vi "Write Sonde Data cells to excel.vi"(0 "NI_report in":refnum<class "NI_report.lvclass">, 1 "milliseconds to wait":u32, 2 "all rows":string[][](array[string]), 3 "Row Offset In":i32=14, 5 "error in (no error)":errorcluster, 6 "Worksheet Names":string[](array[string]), 7 "Sample Array":i32[](array[numeric]), 9 "Sample Row \nBreak points":i32[](array[numeric]), 11 "Number of Sample Sheets":i32) -> (14 "NI_report out":refnum<class "NI_report.lvclass">, 16 "Row Offset Out":i32, 19 "error out":errorcluster)   [LabVIEW 2016]
uses:
  <vilib>/Utility/NIReport.llb/NI_report.lvclass
panel:
  out "Row Offset":i32
  out "sample subarray":string[][](array[string])
  out "Length":i32
  out "Breakpoint size":i32
  out "number of rows":i32
  out "size(s)":i32[](array[numeric])
  out "Current Sample Sheet":string
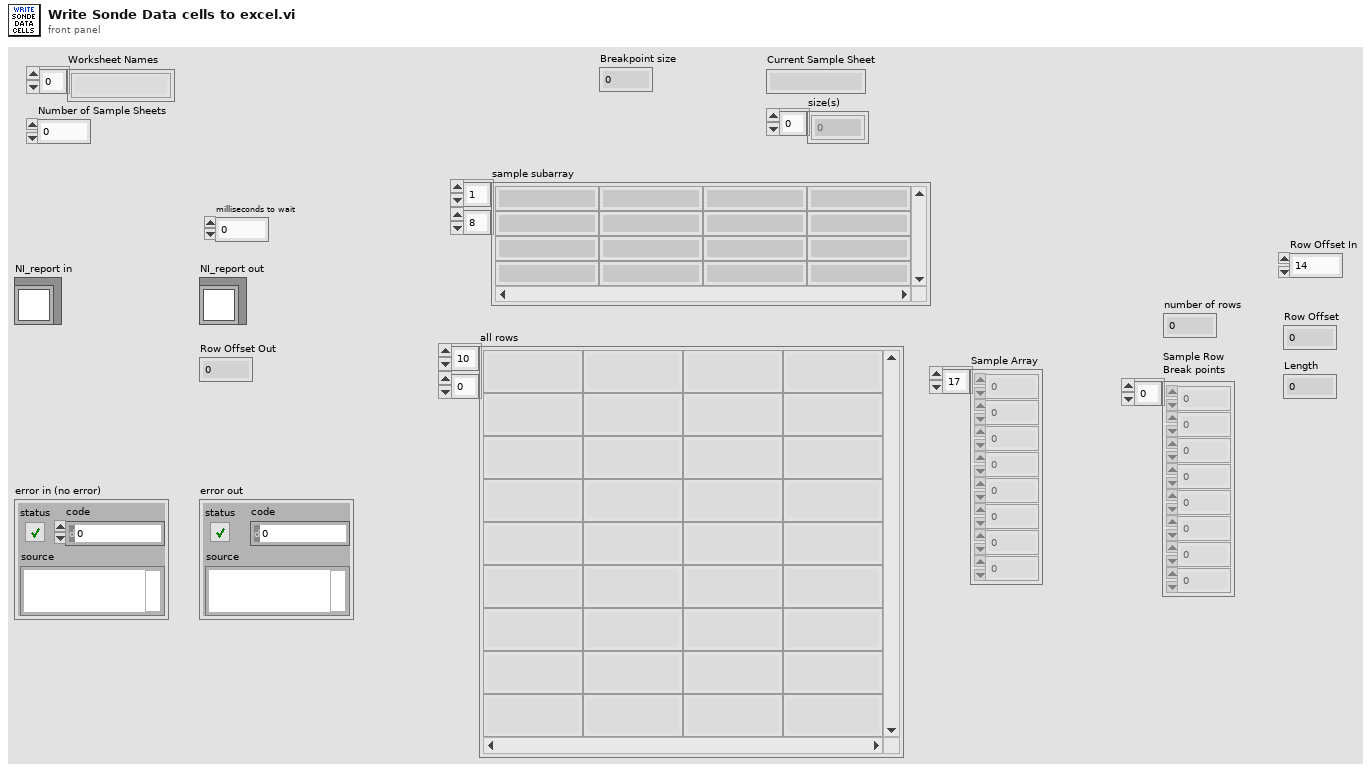
[diagram p1: front panel]
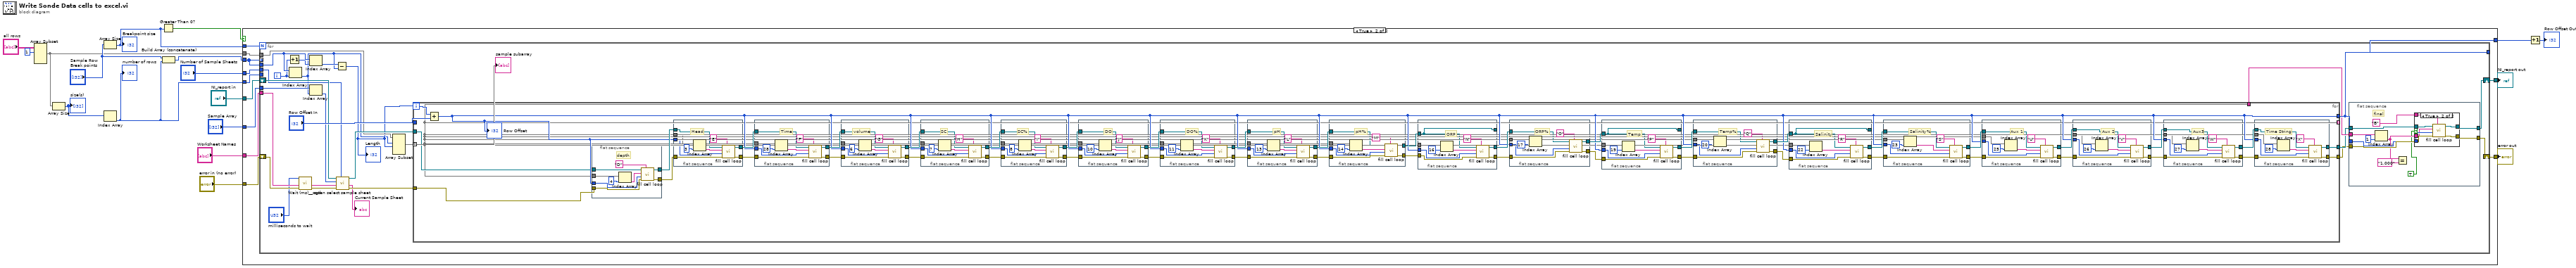
[diagram p0: block diagram]
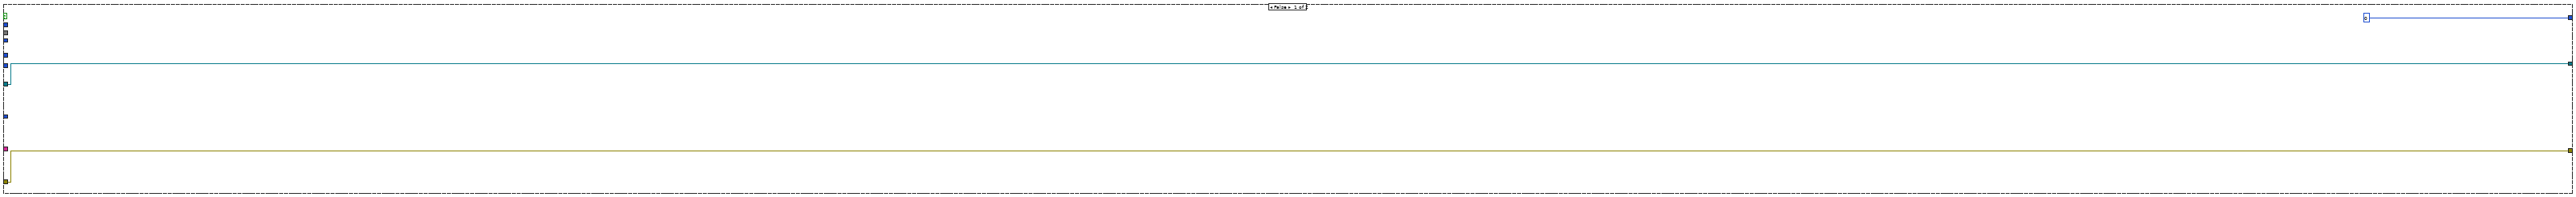
[diagram p2: hidden frame]
diagram:
  n1 = Array Subset(array="all rows", index (row)=1 ("index")) -> (w4:string[][])  [unwired: 3 in]
  n2 = Array Size(array=w4) -> (size(s)=w3:i32[])
  "size(s)" <- w3
  n3 = Array Size(array="Sample Row \nBreak points") -> (size(s)=w11:i32)
  "Breakpoint size" <- w11
  n4 = Index Array(array=w3) -> (element=w1:i32)  [unwired: 1 in]
  "number of rows" <- w1
  n5 = Greater Than 0?(x=w11) -> (x > 0?=w12:bool)
  n6 = Build Array (concatenate)("Sample Row \nBreak points", w1) -> (w2:i32[])
  n7 = case shown="True" w12 {
    tunnel: [w20 w33] -> w18
    tunnel: [w21 w32] -> w17
    tunnel: [0 ("Row Offset In") w31] -> w16
    tunnel: "NI_report in" -> [w21 w30]
    tunnel: "error in (no error)" -> [w20 w29]
    tunnel: w11 -> [_ w28]
    tunnel: w2 -> [_ w23]
    tunnel: "Sample Array" -> [_ w22]
    tunnel: "Worksheet Names" -> [_ w27]
    tunnel: "Number of Sample Sheets" -> [_ w26]
    tunnel: w4 -> [_ w25]
    tunnel: w1 -> [_ w24]
    frame False {
    }
    frame True {
      n8 = for {
        N: w28 -> [_]
        tunnel: [w41] -> w31
        shift-right: [w38] -> w32
        shift-left: w30 -> [w58]
        shift-right: [w36] -> w33
        shift-left: w29 -> [w56]
        tunnel: w23 -> [_] mode=indexing
        tunnel: w23 -> [w51]
        tunnel: w27 -> [w54]
        tunnel: w26 -> [w53]
        tunnel: w25 -> [w48]
        tunnel: w24 -> [_]
        tunnel: w22 -> [w46]
        i -> [w43]
        n9 = Increment(x=w43) -> (x+1=w50:i32)
        n10 = Index Array(array=w51, index=w43) -> (element=w42:i32)
        n11 = call "Wait (ms)__ogtk.vi"("error in (no error)"=w56, "milliseconds to wait"="milliseconds to wait") -> ("error out"=w35:errorcluster)  [unwired: 8 in, 1 out]
        n12 = Index Array(array=w51, index=w50) -> (element=w47:i32)
        n13 = Index Array(array=w46, index=w42) -> (element=w45:i32)
        n14 = Subtract(x=w47, y=w42) -> (x-y=w44:i32)
        "Length" <- w44
        n15 = call "open select sample sheet.vi"("Number of Sample Sheets"=w53, "error in (no error)"=w35, "Worksheet Names"=w54, "input 1"=w45, "NI_report in"=w58) -> ("error out"=w55:errorcluster, "Current Sample Sheet"=→"Current Sample Sheet":string, "NI_report out"=w57:refnum<class "NI_report.lvclass">)  [unwired: 4 in]
        n16 = Array Subset(array=w48, index (row)=w42, length (row)=w44) -> (w49:string[][])  [unwired: 2 in]
        "sample subarray" <- w49
        n17 = for {
          N: w44 -> [_]
          tunnel: w49 -> [w80] mode=indexing
          tunnel: w57 -> [w82]
          tunnel: w55 -> [w81]
          tunnel: [w86] -> w37
          tunnel: [w85] -> w39
          tunnel: [w80] -> _ mode=indexing
          tunnel: "Row Offset In" -> [w125]
          tunnel: [w84] -> w41
          tunnel: [w80] -> w40
          i -> [w83]
          n18 = Add(x=w83, y=w125) -> (x+y=w84:i32)
          "Row Offset" <- w84
          n19 = flat-sequence {
            tunnel: w80 -> [w304]
            tunnel: w81 -> [w303]
            tunnel: [w302] -> w124
            tunnel: w84 -> [w301]
            tunnel: w82 -> [w299]
            tunnel: [w298] -> w123
            frame #0 {
              # "depth"
              n20 = Index Array(array=w304, index=4) -> (element=w300:string)
              n21 = call "fill cell loop.vi"("Column Letter"="D" ("Depth Column Letter"), "error in (no error)"=w303, "Row"=w301, "String"=w300, "NI_report in"=w299) -> ("error out"=w302:errorcluster, "NI_report out"=w298:refnum<class "NI_report.lvclass">)  [unwired: 5 in]
            }
          }
          n22 = flat-sequence {
            tunnel: [w296] -> w121
            tunnel: [w295] -> w122
            tunnel: w80 -> [w291]
            tunnel: w124 -> [w290]
            tunnel: w84 -> [w289]
            tunnel: w123 -> [w288]
            frame #0 {
              # "Head"
              n23 = Index Array(array=w291, index=3) -> (element=w292:string)
              n24 = call "fill cell loop.vi"("Column Letter"="E" ("Head Column Letter"), "error in (no error)"=w290, "Row"=w289, "String"=w292, "NI_report in"=w288) -> ("error out"=w296:errorcluster, "NI_report out"=w295:refnum<class "NI_report.lvclass">)  [unwired: 5 in]
            }
          }
          n25 = flat-sequence {
            tunnel: [w287] -> w119
            tunnel: [w286] -> w120
            tunnel: w80 -> [w282]
            tunnel: w121 -> [w281]
            tunnel: w84 -> [w280]
            tunnel: w122 -> [w279]
            frame #0 {
              # "Time"
              n26 = Index Array(array=w282, index=28) -> (element=w283:string)
              n27 = call "fill cell loop.vi"("Column Letter"="F" ("Head Column Letter"), "error in (no error)"=w281, "Row"=w280, "String"=w283, "NI_report in"=w279) -> ("error out"=w287:errorcluster, "NI_report out"=w286:refnum<class "NI_report.lvclass">)  [unwired: 5 in]
            }
          }
          n28 = flat-sequence {
            tunnel: [w278] -> w117
            tunnel: [w277] -> w118
            tunnel: w80 -> [w273]
            tunnel: w119 -> [w272]
            tunnel: w84 -> [w271]
            tunnel: w120 -> [w270]
            frame #0 {
              # "volume"
              n29 = Index Array(array=w273, index=6) -> (element=w274:string)
              n30 = call "fill cell loop.vi"("Column Letter"="G" ("Head Column Letter"), "error in (no error)"=w272, "Row"=w271, "String"=w274, "NI_report in"=w270) -> ("error out"=w278:errorcluster, "NI_report out"=w277:refnum<class "NI_report.lvclass">)  [unwired: 5 in]
            }
          }
          n31 = flat-sequence {
            tunnel: [w269] -> w115
            tunnel: [w268] -> w116
            tunnel: w80 -> [w264]
            tunnel: w117 -> [w263]
            tunnel: w84 -> [w262]
            tunnel: w118 -> [w261]
            frame #0 {
              # "SC"
              n32 = Index Array(array=w264, index=7) -> (element=w265:string)
              n33 = call "fill cell loop.vi"("Column Letter"="H" ("Head Column Letter"), "error in (no error)"=w263, "Row"=w262, "String"=w265, "NI_report in"=w261) -> ("error out"=w269:errorcluster, "NI_report out"=w268:refnum<class "NI_report.lvclass">)  [unwired: 5 in]
            }
          }
          n34 = flat-sequence {
            tunnel: [w260] -> w111
            tunnel: [w259] -> w112
            tunnel: w80 -> [w255]
            tunnel: w115 -> [w254]
            tunnel: w84 -> [w253]
            tunnel: w116 -> [w252]
            frame #0 {
              # "SC%"
              n35 = Index Array(array=w255, index=8) -> (element=w256:string)
              n36 = call "fill cell loop.vi"("Column Letter"="I" ("Head Column Letter"), "error in (no error)"=w254, "Row"=w253, "String"=w256, "NI_report in"=w252) -> ("error out"=w260:errorcluster, "NI_report out"=w259:refnum<class "NI_report.lvclass">)  [unwired: 5 in]
            }
          }
          n37 = flat-sequence {
            tunnel: [w251] -> w114
            tunnel: [w250] -> w113
            tunnel: w80 -> [w246]
            tunnel: w111 -> [w245]
            tunnel: w84 -> [w244]
            tunnel: w112 -> [w243]
            frame #0 {
              # "DO"
              n38 = Index Array(array=w246, index=10) -> (element=w247:string)
              n39 = call "fill cell loop.vi"("Column Letter"="J" ("Head Column Letter"), "error in (no error)"=w245, "Row"=w244, "String"=w247, "NI_report in"=w243) -> ("error out"=w251:errorcluster, "NI_report out"=w250:refnum<class "NI_report.lvclass">)  [unwired: 5 in]
            }
          }
          n40 = flat-sequence {
            tunnel: [w242] -> w107
            tunnel: [w241] -> w108
            tunnel: w80 -> [w237]
            tunnel: w114 -> [w236]
            tunnel: w84 -> [w235]
            tunnel: w113 -> [w234]
            frame #0 {
              # "DO%"
              n41 = Index Array(array=w237, index=11) -> (element=w238:string)
              n42 = call "fill cell loop.vi"("Column Letter"="K" ("Head Column Letter"), "error in (no error)"=w236, "Row"=w235, "String"=w238, "NI_report in"=w234) -> ("error out"=w242:errorcluster, "NI_report out"=w241:refnum<class "NI_report.lvclass">)  [unwired: 5 in]
            }
          }
          n43 = flat-sequence {
            tunnel: [w233] -> w109
            tunnel: [w232] -> w110
            tunnel: w80 -> [w228]
            tunnel: w107 -> [w227]
            tunnel: w84 -> [w226]
            tunnel: w108 -> [w225]
            frame #0 {
              # "pH"
              n44 = Index Array(array=w228, index=13) -> (element=w229:string)
              n45 = call "fill cell loop.vi"("Column Letter"="L" ("Head Column Letter"), "error in (no error)"=w227, "Row"=w226, "String"=w229, "NI_report in"=w225) -> ("error out"=w233:errorcluster, "NI_report out"=w232:refnum<class "NI_report.lvclass">)  [unwired: 5 in]
            }
          }
          n46 = flat-sequence {
            tunnel: [w224] -> w104
            tunnel: [w223] -> w103
            tunnel: w80 -> [w219]
            tunnel: w109 -> [w218]
            tunnel: w84 -> [w217]
            tunnel: w110 -> [w216]
            frame #0 {
              # "pH%"
              n47 = Index Array(array=w219, index=14) -> (element=w220:string)
              n48 = call "fill cell loop.vi"("Column Letter"="M" ("Head Column Letter"), "error in (no error)"=w218, "Row"=w217, "String"=w220, "NI_report in"=w216) -> ("error out"=w224:errorcluster, "NI_report out"=w223:refnum<class "NI_report.lvclass">)  [unwired: 5 in]
            }
          }
          n49 = flat-sequence {
            tunnel: [w215] -> w106
            tunnel: [w214] -> w105
            tunnel: w80 -> [w210]
            tunnel: w104 -> [w209]
            tunnel: w84 -> [w208]
            tunnel: [w207] -> _
            tunnel: w103 -> [w207]
            frame #0 {
              # "ORP"
              n50 = Index Array(array=w210, index=16) -> (element=w211:string)
              n51 = call "fill cell loop.vi"("Column Letter"="N" ("Head Column Letter"), "error in (no error)"=w209, "Row"=w208, "String"=w211, "NI_report in"=w207) -> ("error out"=w215:errorcluster, "NI_report out"=w214:refnum<class "NI_report.lvclass">)  [unwired: 5 in]
            }
          }
          n52 = flat-sequence {
            tunnel: [w206] -> w100
            tunnel: [w205] -> w99
            tunnel: w80 -> [w201]
            tunnel: w106 -> [w200]
            tunnel: w84 -> [w199]
            tunnel: w105 -> [w198]
            frame #0 {
              # "ORP%"
              n53 = Index Array(array=w201, index=17) -> (element=w202:string)
              n54 = call "fill cell loop.vi"("Column Letter"="O" ("Head Column Letter"), "error in (no error)"=w200, "Row"=w199, "String"=w202, "NI_report in"=w198) -> ("error out"=w206:errorcluster, "NI_report out"=w205:refnum<class "NI_report.lvclass">)  [unwired: 5 in]
            }
          }
          n55 = flat-sequence {
            tunnel: [w179] -> w96
            tunnel: [w178] -> w95
            tunnel: w80 -> [w174]
            tunnel: w100 -> [w173]
            tunnel: w84 -> [w172]
            tunnel: w99 -> [w171]
            tunnel: [w171] -> _
            frame #0 {
              # "Temp"
              n56 = Index Array(array=w174, index=19) -> (element=w175:string)
              n57 = call "fill cell loop.vi"("Column Letter"="P" ("Head Column Letter"), "error in (no error)"=w173, "Row"=w172, "String"=w175, "NI_report in"=w171) -> ("error out"=w179:errorcluster, "NI_report out"=w178:refnum<class "NI_report.lvclass">)  [unwired: 5 in]
            }
          }
          n58 = flat-sequence {
            tunnel: [w170] -> w97
            tunnel: [w169] -> w98
            tunnel: w80 -> [w165]
            tunnel: w84 -> [w164]
            tunnel: w96 -> [w163]
            tunnel: w95 -> [w162]
            frame #0 {
              # "Temp%"
              n59 = Index Array(array=w165, index=20) -> (element=w166:string)
              n60 = call "fill cell loop.vi"("Column Letter"="Q" ("Head Column Letter"), "error in (no error)"=w163, "Row"=w164, "String"=w166, "NI_report in"=w162) -> ("error out"=w170:errorcluster, "NI_report out"=w169:refnum<class "NI_report.lvclass">)  [unwired: 5 in]
            }
          }
          n61 = flat-sequence {
            tunnel: [w197] -> w101
            tunnel: [w196] -> w102
            tunnel: w80 -> [w192]
            tunnel: w97 -> [w191]
            tunnel: w84 -> [w190]
            tunnel: w98 -> [w189]
            tunnel: [w189] -> _
            frame #0 {
              # "Salinity"
              n62 = Index Array(array=w192, index=22) -> (element=w193:string)
              n63 = call "fill cell loop.vi"("Column Letter"="R" ("Head Column Letter"), "error in (no error)"=w191, "Row"=w190, "String"=w193, "NI_report in"=w189) -> ("error out"=w197:errorcluster, "NI_report out"=w196:refnum<class "NI_report.lvclass">)  [unwired: 5 in]
            }
          }
          n64 = flat-sequence {
            tunnel: [w188] -> w93
            tunnel: [w187] -> w94
            tunnel: w80 -> [w183]
            tunnel: w101 -> [w182]
            tunnel: w84 -> [w181]
            tunnel: w102 -> [w180]
            frame #0 {
              # "Salinity%"
              n65 = Index Array(array=w183, index=23) -> (element=w184:string)
              n66 = call "fill cell loop.vi"("Column Letter"="S" ("Head Column Letter"), "error in (no error)"=w182, "Row"=w181, "String"=w184, "NI_report in"=w180) -> ("error out"=w188:errorcluster, "NI_report out"=w187:refnum<class "NI_report.lvclass">)  [unwired: 5 in]
            }
          }
          n67 = flat-sequence {
            tunnel: [w161] -> w91
            tunnel: [w160] -> w92
            tunnel: w80 -> [w156]
            tunnel: w93 -> [w155]
            tunnel: w84 -> [w154]
            tunnel: w94 -> [w153]
            frame #0 {
              # "Aux 1"
              n68 = Index Array(array=w156, index=25) -> (element=w157:string)
              n69 = call "fill cell loop.vi"("Column Letter"="U" ("Head Column Letter"), "error in (no error)"=w155, "Row"=w154, "String"=w157, "NI_report in"=w153) -> ("error out"=w161:errorcluster, "NI_report out"=w160:refnum<class "NI_report.lvclass">)  [unwired: 5 in]
            }
          }
          n70 = flat-sequence {
            tunnel: [w152] -> w90
            tunnel: [w151] -> w89
            tunnel: w80 -> [w147]
            tunnel: w91 -> [w146]
            tunnel: w84 -> [w145]
            tunnel: w92 -> [w144]
            frame #0 {
              # "Aux 2"
              n71 = Index Array(array=w147, index=26) -> (element=w148:string)
              n72 = call "fill cell loop.vi"("Column Letter"="V" ("Head Column Letter"), "error in (no error)"=w146, "Row"=w145, "String"=w148, "NI_report in"=w144) -> ("error out"=w152:errorcluster, "NI_report out"=w151:refnum<class "NI_report.lvclass">)  [unwired: 5 in]
            }
          }
          n73 = flat-sequence {
            tunnel: [w143] -> w87
            tunnel: [w142] -> w88
            tunnel: w80 -> [w138]
            tunnel: w90 -> [w137]
            tunnel: w84 -> [w136]
            tunnel: w89 -> [w135]
            frame #0 {
              # "Aux3"
              n74 = Index Array(array=w138, index=27) -> (element=w139:string)
              n75 = call "fill cell loop.vi"("Column Letter"="W" ("Head Column Letter"), "error in (no error)"=w137, "Row"=w136, "String"=w139, "NI_report in"=w135) -> ("error out"=w143:errorcluster, "NI_report out"=w142:refnum<class "NI_report.lvclass">)  [unwired: 5 in]
            }
          }
          n76 = flat-sequence {
            tunnel: [w134] -> w86
            tunnel: [w133] -> w85
            tunnel: w80 -> [w129]
            tunnel: w87 -> [w128]
            tunnel: w84 -> [w127]
            tunnel: w88 -> [w126]
            frame #0 {
              # "Time String"
              n77 = Index Array(array=w129, index=28) -> (element=w130:string)
              n78 = call "fill cell loop.vi"("Column Letter"="X" ("Head Column Letter"), "error in (no error)"=w128, "Row"=w127, "String"=w130, "NI_report in"=w126) -> ("error out"=w134:errorcluster, "NI_report out"=w133:refnum<class "NI_report.lvclass">)  [unwired: 5 in]
            }
          }
        }
        n79 = flat-sequence {
          tunnel: w40 -> [w69]
          tunnel: w37 -> [w68]
          tunnel: [w67] -> w36
          tunnel: w41 -> [w66]
          tunnel: w39 -> [w65]
          tunnel: [w64] -> w38
          frame #0 {
            # "final"
            n80 = Index Array(array=w69, index=1) -> (element=w62:string)
            n81 = Equal?(x=w62, y="1.000") -> ()  [unwired: 1 out]
            n82 = case shown="True" TRUE {
              tunnel: w68 -> [w71 w79]
              tunnel: [w71 w78] -> w67
              tunnel: w66 -> [_ w77]
              tunnel: w62 -> [_ w76]
              tunnel: w65 -> [w72 w75]
              tunnel: [w72 w74] -> w64
              tunnel: "B" ("Depth Column Letter") -> [_ w73]
              frame False {
              }
              frame True {
                n83 = call "fill cell loop.vi"("Column Letter"=w73, "error in (no error)"=w79, "Row"=w77, "String"=w76, "NI_report in"=w75) -> ("error out"=w78:errorcluster, "NI_report out"=w74:refnum<class "NI_report.lvclass">)  [unwired: 5 in]
              }
            }
          }
        }
      }
    }
  }
  "error out" <- w18
  "NI_report out" <- w17
  n84 = Increment(x=w16) -> (x+1=→"Row Offset Out":i32)
